vi "Dispense FN - OFF - Timer (SubVI).vi"(0 "Settings 2":T1={"ON Settings"={"Enable Dynamic Setpoint?"=TRUE, "Enable Dynamic Dispense Time?"=TRUE, "Enable Drain Rate Functions"=TRUE, "Dispense Sample Time (s)"=0.5, "Dispense Slope Ave"=0, "ON Timeout (sec)"=600.0, "1st Setpoint (% of Target)"=0.0, "2nd Setpoint (% of Target)"=0.0, "3rd Setpoint (% of Target)"=0.0, "Measure Dispense Delay (sec)"=0.0, "Settle Slope Sample Time (s)"=0.0}, "OFF Settings"={"Drain Sample Time (s)"=0.5, "Drain Rate Ave Size"=5, "Drain Rate Limits (± g/sec)"=10.0, "Level Slope Range (± g/sec)"=0.25, "OFF Timeout (sec)"=0.0, "Near SP Slope Level (± g/sec)"=0.01, "Near Setpoint Threshold (%)"=95.0}, "Overshoot Settings"={"Time Limit (s)"=60.0, "Container MAX (g)"=1500.0, "Max FILL Slope (+/- g/sec)"=10.0, "% Overshot to Enable (>)"=0.25}, "FILL Timeout (s)"=300.0, "Full Settle Time (s)"=3.0, "Pre-Hydrate \nSpray Time (s)"=10.0, "Pre-Hydrate \nWait Time (s)"=30.0}, 5 "Reset":bool) -> (14 "Sample":bool, 16 "Max Drain Complete?":bool, 19 "Elapsed Time (s)":dbl)   [LabVIEW 2009]
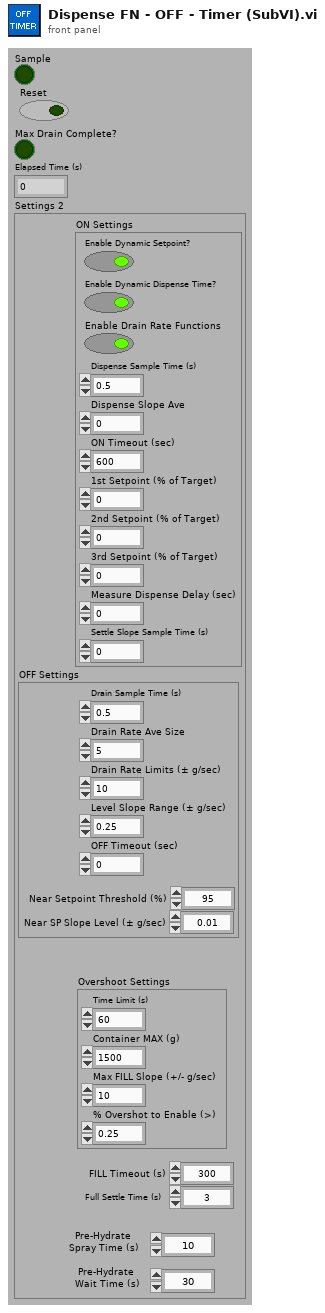
[diagram p1: front panel]
types:
  T1 = cluster{"ON Settings":cluster{"Enable Dynamic Setpoint?":bool, "Enable Dynamic Dispense Time?":bool, "Enable Drain Rate Functions":bool, "Dispense Sample Time (s)":dbl, "Dispense Slope Ave":i32, "ON Timeout (sec)":dbl, "1st Setpoint (% of Target)":dbl, "2nd Setpoint (% of Target)":dbl, "3rd Setpoint (% of Target)":dbl, "Measure Dispense Delay (sec)":dbl, "Settle Slope Sample Time (s)":dbl}, "OFF Settings":cluster{"Drain Sample Time (s)":dbl, "Drain Rate Ave Size":i32, "Drain Rate Limits (± g/sec)":dbl, "Level Slope Range (± g/sec)":dbl, "OFF Timeout (sec)":dbl, "Near SP Slope Level (± g/sec)":dbl, "Near Setpoint Threshold (%)":dbl}, "Overshoot Settings":cluster{"Time Limit (s)":dbl, "Container MAX (g)":dbl, "Max FILL Slope (+/- g/sec)":dbl, "% Overshot to Enable (>)":dbl}, "FILL Timeout (s)":dbl, "Full Settle Time (s)":dbl, "Pre-Hydrate \nSpray Time (s)":dbl, "Pre-Hydrate \nWait Time (s)":dbl}
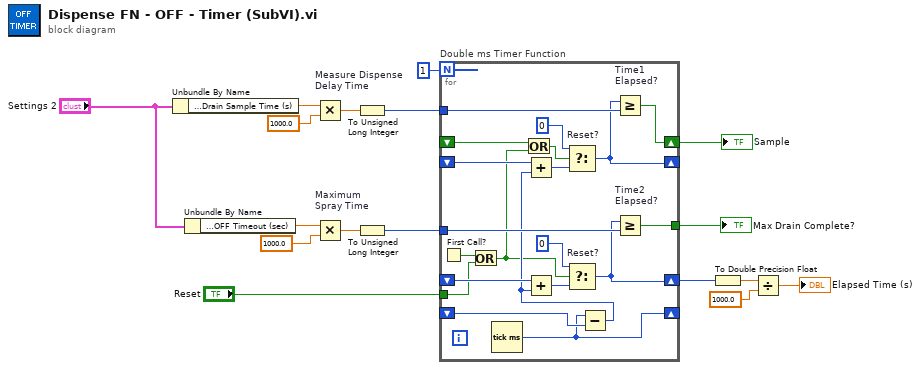
[diagram p0: block diagram]
diagram:
  n1 = Unbundle By Name("Settings 2") -> ("OFF Settings.Drain Sample Time (s)"=w13:dbl)
  n2 = Unbundle By Name("Settings 2") -> ("OFF Settings.OFF Timeout (sec)"=w12:dbl)
  n3 = Multiply "Measure Dispense\nDelay Time"(x=w13, y=1000.0) -> (x*y=w8:dbl)
  n4 = Multiply "Maximum\nSpray Time"(x=w12, y=1000.0) -> (x*y=w5:dbl)
  n5 = To Unsigned Long Integer(number=w8) -> (unsigned 32bit integer=w7:u32)
  n6 = To Unsigned Long Integer(number=w5) -> (unsigned 32bit integer=w4:u32)
  n7 = for "Double ms Timer Function" {
    N: 1 -> [_]
    shift-right: [w36] -> _
    shift-left: _ -> [w37]
    tunnel: w7 -> [w34]
    shift-right: [w28] -> w2
    shift-left: _ -> [w31]
    tunnel: w4 -> [w30]
    tunnel: [w29] -> w15
    tunnel: "Reset" -> [w26]
    shift-right: [w18] -> _
    shift-left: _ -> [w22]
    shift-right: [w35] -> w14
    shift-left: _ -> [w19]
    n8 = First Call?() -> (First Call?: T/F=w27:bool)
    n9 = Or(x=w27, y=w26) -> (x .or. y?=w21:bool)
    n10 = Tick Count (ms)() -> (millisecond timer value=w36:u32)
    n11 = Or(x=w19, y=w21) -> (x .or. y?=w20:bool)
    n12 = Subtract(x=w36, y=w37) -> (x-y=w23:u32)
    n13 = Add(x=w22, y=w23) -> (x+y=w25:u32)
    n14 = Add(x=w31, y=w23) -> (x+y=w33:u32)
    n15 = Select "Reset?"(t=u32 0, s=w20, f=w25) -> (s? t:f=w18:u32)
    n16 = Select "Reset?"(t=u32 0, s=w21, f=w33) -> (s? t:f=w28:u32)
    n17 = Greater Or Equal? "Time1\nElapsed?"(x=w18, y=w34) -> (x >= y?=w35:bool)
    n18 = Greater Or Equal? "Time2\nElapsed?"(x=w28, y=w30) -> (x >= y?=w29:bool)
  }
  "Max Drain Complete?" <- w15
  "Sample" <- w14
  n19 = To Double Precision Float(number=w2) -> (double precision float=w3:dbl)
  n20 = Divide(x=w3, y=1000.0) -> (x/y=→"Elapsed Time (s)":dbl)
